vi "workbook add vba project.vi"(8 "error in (no error)":errorcluster, 10 "filename":string, 11 "workbook":u32) -> (0 "error out":errorcluster, 3 "function return":u32(ring))   [LabVIEW 8.6]
doc: "lxw_error workbook_add_vba_project(lxw_workbook workbook, const char *filename);"
uses:
  pending_lvxlsxwriter/xlsxwriter.dll
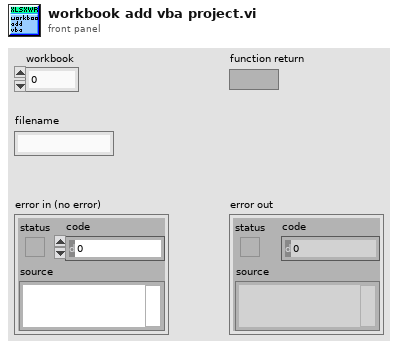
[diagram p1: front panel]
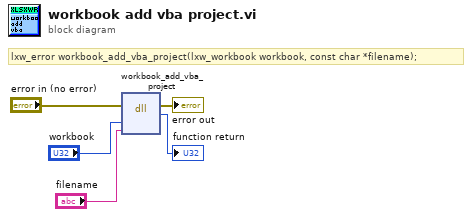
[diagram p0: block diagram]
diagram:
  # "lxw_error workbook_add_vba_project(lxw_workbook workbook, const char *filename);"
  n1 = dll-call lib="C:/Users/WDAGUtilityAccount/Desktop/pending_lvxlsxwriter/xlsxwriter.*" fn="workbook_add_vba_project"(error in="error in (no error)", "workbook"="workbook", "filename"="filename") -> (error out=→"error out":errorcluster, →"function return":u32)  [unwired: 4 in, 1 out]
